vi "Read Matlab Params.vi"(8 "error in (no error)":errorcluster, 10 "Enum":T1(ring), 11 "TrialBasedExperiment in":refnum<class "FleTraining.lvclass">) -> (0 "error out":errorcluster, 2 "Matlab Param Array":cluster{"Name":string, "Data":variant}[](array[cluster]), 3 "TrialBasedExperiment out":refnum<class "FleTraining.lvclass">)   [LabVIEW 2014, in "FleTraining.lvclass"]
uses:
  FleTraining.lvclass
  FleTraining.lvclass/FleTraining.ctl
  TwoAfcEye/TwoAfcEye.lvclass
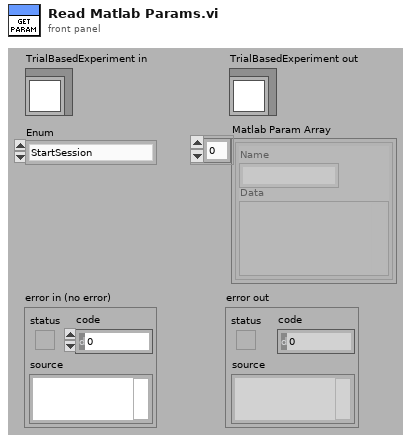
[diagram p1: front panel]
types:
  T1 = enum16{"StartSession", "StartTrial", "ShowStimulus"}
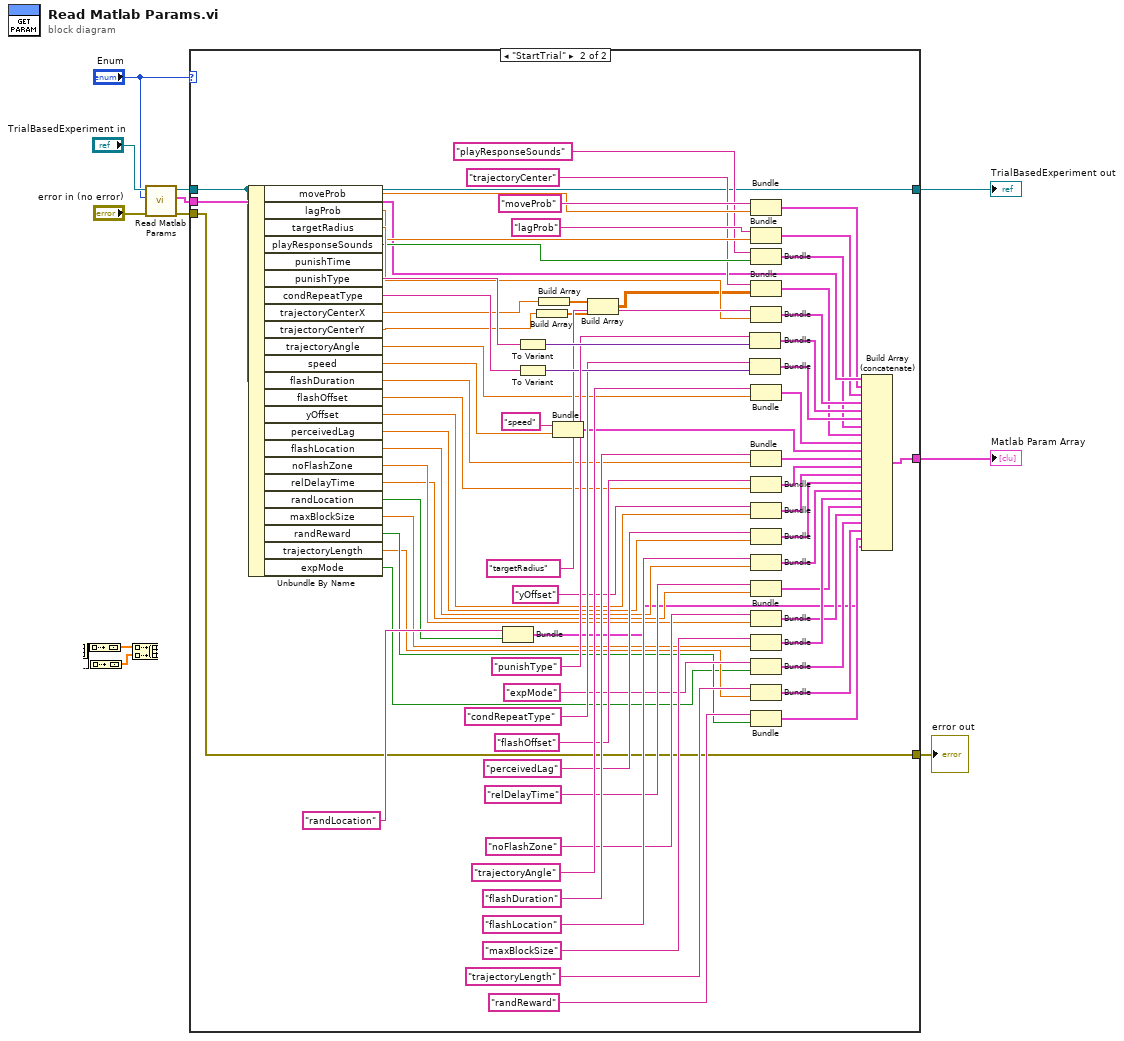
[diagram p0: block diagram]
diagram:
  n1 = call-parent "Read Matlab Params.vi"("error in (no error)"="error in (no error)", "Enum"="Enum", "TrialBasedExperiment in"="TrialBasedExperiment in") -> ("error out"=w2:errorcluster, "Matlab Param Array"=w6:cluster{"Name":string, "Data":variant}[], "TrialBasedExperiment out"=w7:refnum<class "FleTraining.lvclass">)  [unwired: 6 in]
  n2 = case shown="\"StartTrial\"" "Enum" {
    tunnel: w7 -> [w11 w20]
    tunnel: w6 -> [w12 w42]
    tunnel: [w12 w21] -> w5
    tunnel: [w11 w20] -> w3
    tunnel: w2 -> [w10 w19]
    tunnel: [w10 w19] -> w1
    frame "StartSession", Default {
    }
    frame "StartTrial" {
      n3 = Unbundle By Name(w20) -> ("moveProb"=w78:dbl, "lagProb"=w74:dbl, "targetRadius"=w75:dbl, "playResponseSounds"=w72:bool, "punishType"=w85:string, "condRepeatType"=w82:string, "trajectoryCenterX"=w17:dbl, "trajectoryCenterY"=w16:dbl, "trajectoryAngle"=w56:dbl, "speed"=w55:dbl, "flashDuration"=w54:dbl, "flashOffset"=w53:dbl, "yOffset"=w52:dbl, "perceivedLag"=w51:dbl, "flashLocation"=w50:dbl, "noFlashZone"=w49:dbl, "relDelayTime"=w48:dbl, "randLocation"=w47:bool, "maxBlockSize"=w46:dbl, "randReward"=w45:bool, "trajectoryLength"=w44:dbl, "expMode"=w43:bool)  [unwired: 1 out]
      n4 = Bundle("randLocation", "randLocation"=w47) -> (w18:cluster{string, "randLocation":bool})  [unwired: 1 out]
      n5 = To Variant(anything=w85) -> (Variant=w84:variant)
      n6 = To Variant(anything=w82) -> (Variant=w81:variant)
      n7 = Build Array(w16) -> (w14:dbl[])
      n8 = Build Array(w17) -> (w15:dbl[])
      n9 = Bundle("speed", "speed"=w55) -> (w33:cluster{string, "speed":dbl})  [unwired: 1 out]
      n10 = Build Array(w15, w14) -> (w13:dbl[][])
      n11 = Bundle("punishType", "Variant"=w84) -> (w38:cluster{string, "Variant":variant})  [unwired: 1 out]
      n12 = Bundle("condRepeatType", "Variant"=w81) -> (w37:cluster{string, "Variant":variant})  [unwired: 1 out]
      n13 = Bundle("moveProb", "moveProb"=w78) -> (w41:cluster{string, "moveProb":dbl})  [unwired: 1 out]
      n14 = Bundle("lagProb", "lagProb"=w74) -> (w40:cluster{string, "lagProb":dbl})  [unwired: 1 out]
      n15 = Bundle("playResponseSounds", "playResponseSounds"=w72) -> (w36:cluster{string, "playResponseSounds":bool})  [unwired: 1 out]
      n16 = Bundle("trajectoryCenter", w13) -> (w35:cluster{string, dbl[][]})  [unwired: 1 in]
      n17 = Bundle("targetRadius", "targetRadius"=w75) -> (w39:cluster{string, "targetRadius":dbl})  [unwired: 1 out]
      n18 = Bundle("trajectoryAngle", "trajectoryAngle"=w56) -> (w34:cluster{string, "trajectoryAngle":dbl})  [unwired: 1 out]
      n19 = Bundle("flashDuration", "flashDuration"=w54) -> (w32:cluster{string, "flashDuration":dbl})  [unwired: 1 out]
      n20 = Bundle("flashOffset", "flashOffset"=w53) -> (w31:cluster{string, "flashOffset":dbl})  [unwired: 1 out]
      n21 = Bundle("yOffset", "yOffset"=w52) -> (w30:cluster{string, "yOffset":dbl})  [unwired: 1 out]
      n22 = Bundle("perceivedLag", "perceivedLag"=w51) -> (w29:cluster{string, "perceivedLag":dbl})  [unwired: 1 out]
      n23 = Bundle("flashLocation", "flashLocation"=w50) -> (w28:cluster{string, "flashLocation":dbl})  [unwired: 1 out]
      n24 = Bundle("relDelayTime", "relDelayTime"=w48) -> (w26:cluster{string, "relDelayTime":dbl})  [unwired: 1 out]
      n25 = Bundle("noFlashZone", "noFlashZone"=w49) -> (w25:cluster{string, "noFlashZone":dbl})  [unwired: 1 out]
      n26 = Bundle("maxBlockSize", "maxBlockSize"=w46) -> (w27:cluster{string, "maxBlockSize":dbl})  [unwired: 1 out]
      n27 = Bundle("expMode", "expMode"=w43) -> (w24:cluster{string, "expMode":bool})  [unwired: 1 out]
      n28 = Bundle("trajectoryLength", "trajectoryLength"=w44) -> (w23:cluster{string, "trajectoryLength":dbl})  [unwired: 1 out]
      n29 = Bundle("randReward", "randReward"=w45) -> (w22:cluster{string, "randReward":bool})  [unwired: 1 out]
      n30 = Build Array (concatenate)(w42, w41, w40, w39, w38, w37, w36, w35, w34, w33, w32, w31, w30, w29, w28, w27, w26, w25, w24, w23, w22, w18) -> (w21:cluster{"Name":string, "Variant":variant}[])
    }
  }
  "error out" <- w1
  "TrialBasedExperiment out" <- w3
  "Matlab Param Array" <- w5
